vi "Multi-socket save data.vi"(0 "TMN DC\\CAP Data Log File Path":path=path "C:/temp", 1 "SN":T2={"SN_S1"="01", "SN_S2"="02", "SN_S3"="03", "SN_S4"="04", "SN_S5"="05", "SN_S6"="06", "SN_S7"="07", "SN_S8"="08", "SN_S9"="09", "SN_S10"="10", "SN_S11"="11", "SN_S12"="12", "SN_S13"="13", "SN_S14"="14", "SN_S15"="15", "SN_S16"="16"}, 2 "EFUSE":T1={"S1_EFUSE"="0", "S2_EFUSE"="01", "S3_EFUSE"="02", "S4_EFUSE"="04", "S5_EFUSE"="05", "S6_EFUSE"="06", "S7_EFUSE"="07", "S8_EFUSE"="08", "S9_EFUSE"="09", "S10_EFUSE"="10", "S11_EFUSE"="11", "S12_EFUSE"="12", "S13_EFUSE"="13", "S14_EFUSE"="14", "S15_EFUSE"="15", "S16_EFUSE"="16"}, 3 "Lot#":string="WS1033", 4 "Wafer#":string="T4", 5 "File Name":string="Test Data", 7 "error in":errorcluster, 8 "Multi Socket Data Out":string[][](array[string])=[["1", "1", "1", "1", "1", "1", "1", "1", "1", "1", "1", "1", "1", "1", "1", "1", "1", "1", "1", "1", "1", "1", "1", "1", "1", "1", "1", "1", "1", "1", "1", "1", "1", "1", "1", "1", "1", "1", "1", "1", "1", "1", "1", "1", "1", "1", "1", "1", "1", "1", "1", "1", "1", "1", "1", "1", "1", "1", "1", "1", "1", "1", "1", "1", "1", "1", "1", "1", "1", "1", "1", "1", "1", "1", "1", "1", "1", "1", "1", "1", "1", "1", "1"], ["2", "2", "2", "2", "2", "2", "2", "2", "2", "2", "2", "2", "2", "2", "2", "2", "2", "2", "2", "2", "2", "2", "2", "2", "2", "2", "2", "2", "2", "2", "2", "2", "2", "2", "2", "2", "2", "2", "2", "2", "2", "2", "2", "2", "2", "2", "2", "2", "2", "2", "2", "2", "2", "2", "2", "2", "2", "2", "2", "2", "2", "2", "2", "2", "2", "2", "2", "2", "2", "2", "2", "2", "2", "2", "2", "2", "2", "2", "2", "2", "2", "2", "2"], ["3", "3", "3", "3", "3", "3", "3", "3", "3", "3", "3", "3", "3", "3", "3", "3", "3", "3", "3", "3", "3", "3", "3", "3", "3", "3", "3", "3", "3", "3", "3", "3", "3", "3", "3", "3", "3", "3", "3", "3", "3", "3", "3", "3", "3", "3", "3", "3", "3", "3", "3", "3", "3", "3", "3", "3", "3", "3", "3", "3", "3", "3", "3", "3", "3", "3", "3", "3", "3", "3", "3", "3", "3", "3", "3", "3", "3", "3", "3", "3", "3", "3", "3"], ["4", "4", "4", "4", "4", "4", "4", "4", "4", "4", "4", "4", "4", "4", "4", "4", "4", "4", "4", "4", "4", "4", "4", "4", "4", "4", "4", "4", "4", "4", "4", "4", "4", "4", "4", "4", "4", "4", "4", "4", "4", "4", "4", "4", "4", "4", "4", "4", "4", "4", "4", "4", "4", "4", "4", "4", "4", "4", "4", "4", "4", "4", "4", "4", "4", "4", "4", "4", "4", "4", "4", "4", "4", "4", "4", "4", "4", "4", "4", "4", "4", "4", "4"], ["5", "5", "5", "5", "5", "5", "5", "5", "5", "5", "5", "5", "5", "5", "5", "5", "5", "5", "5", "5", "5", "5", "5", "5", "5", "5", "5", "5", "5", "5", "5", "5", "5", "5", "5", "5", "5", "5", "5", "5", "5", "5", "5", "5", "5", "5", "5", "5", "5", "5", "5", "5", "5", "5", "5", "5", "5", "5", "5", "5", "5", "5", "5", "5", "5", "5", "5", "5", "5", "5", "5", "5", "5", "5", "5", "5", "5", "5", "5", "5", "5", "5", "5"], ["6", "6", "6", "6", "6", "6", "6", "6", "6", "6", "6", "6", "6", "6", "6", "6", "6", "6", "6", "6", "6", "6", "6", "6", "6", "6", "6", "6", "6", "6", "6", "6", "6", "6", "6", "6", "6", "6", "6", "6", "6", "6", "6", "6", "6", "6", "6", "6", "6", "6", "6", "6", "6", "6", "6", "6", "6", "6", "6", "6", "6", "6", "6", "6", "6", "6", "6", "6", "6", "6", "6", "6", "6", "6", "6", "6", "6", "6", "6", "6", "6", "6", "6"], ["7", "7", "7", "7", "7", "7", "7", "7", "7", "7", "7", "7", "7", "7", "7", "7", "7", "7", "7", "7", "7", "7", "7", "7", "7", "7", "7", "7", "7", "7", "7", "7", "7", "7", "7", "7", "7", "7", "7", "7", "7", "7", "7", "7", "7", "7", "7", "7", "7", "7", "7", "7", "7", "7", "7", "7", "7", "7", "7", "7", "7", "7", "7", "7", "7", "7", "7", "7", "7", "7", "7", "7", "7", "7", "7", "7", "7", "7", "7", "7", "7", "7", "7"], ["8", "8", "8", "8", "8", "8", "8", "8", "8", "8", "8", "8", "8", "8", "8", "8", "8", "8", "8", "8", "8", "8", "8", "8", "8", "8", "8", "8", "8", "8", "8", "8", "8", "8", "8", "8", "8", "8", "8", "8", "8", "8", "8", "8", "8", "8", "8", "8", "8", "8", "8", "8", "8", "8", "8", "8", "8", "8", "8", "8", "8", "8", "8", "8", "8", "8", "8", "8", "8", "8", "8", "8", "8", "8", "8", "8", "8", "8", "8", "8", "8", "8", "8"], ["9", "9", "9", "9", "9", "9", "9", "9", "9", "9", "9", "9", "9", "9", "9", "9", "9", "9", "9", "9", "9", "9", "9", "9", "9", "9", "9", "9", "9", "9", "9", "9", "9", "9", "9", "9", "9", "9", "9", "9", "9", "9", "9", "9", "9", "9", "9", "9", "9", "9", "9", "9", "9", "9", "9", "9", "9", "9", "9", "9", "9", "9", "9", "9", "9", "9", "9", "9", "9", "9", "9", "9", "9", "9", "9", "9", "9", "9", "9", "9", "9", "9", "9"], ["10", "10", "10", "10", "10", "10", "10", "10", "10", "10", "10", "10", "10", "10", "10", "10", "10", "10", "10", "10", "10", "10", "10", "10", "10", "10", "10", "10", "10", "10", "10", "10", "10", "10", "10", "10", "10", "10", "10", "10", "10", "10", "10", "10", "10", "10", "10", "10", "10", "10", "10", "10", "10", "10", "10", "10", "10", "10", "10", "10", "10", "10", "10", "10", "10", "10", "10", "10", "10", "10", "10", "10", "10", "10", "10", "10", "10", "10", "10", "10", "10", "10", "10"], ["11", "11", "11", "11", "11", "11", "11", "11", "11", "11", "11", "11", "11", "11", "11", "11", "11", "11", "11", "11", "11", "11", "11", "11", "11", "11", "11", "11", "11", "11", "11", "11", "11", "11", "11", "11", "11", "11", "11", "11", "11", "11", "11", "11", "11", "11", "11", "11", "11", "11", "11", "11", "11", "11", "11", "11", "11", "11", "11", "11", "11", "11", "11", "11", "11", "11", "11", "11", "11", "11", "11", "11", "11", "11", "11", "11", "11", "11", "11", "11", "11", "11", "11"], ["12", "12", "12", "12", "12", "12", "12", "12", "12", "12", "12", "12", "12", "12", "12", "12", "12", "12", "12", "12", "12", "12", "12", "12", "12", "12", "12", "12", "12", "12", "12", "12", "12", "12", "12", "12", "12", "12", "12", "12", "12", "12", "12", "12", "12", "12", "12", "12", "12", "12", "12", "12", "12", "12", "12", "12", "12", "12", "12", "12", "12", "12", "12", "12", "12", "12", "12", "12", "12", "12", "12", "12", "12", "12", "12", "12", "12", "12", "12", "12", "12", "12", "12"], ["13", "13", "13", "13", "13", "13", "13", "13", "13", "13", "13", "13", "13", "13", "13", "13", "13", "13", "13", "13", "13", "13", "13", "13", "13", "13", "13", "13", "13", "13", "13", "13", "13", "13", "13", "13", "13", "13", "13", "13", "13", "13", "13", "13", "13", "13", "13", "13", "13", "13", "13", "13", "13", "13", "13", "13", "13", "13", "13", "13", "13", "13", "13", "13", "13", "13", "13", "13", "13", "13", "13", "13", "13", "13", "13", "13", "13", "13", "13", "13", "13", "13", "13"], ["14", "14", "14", "14", "14", "14", "14", "14", "14", "14", "14", "14", "14", "14", "14", "14", "14", "14", "14", "14", "14", "14", "14", "14", "14", "14", "14", "14", "14", "14", "14", "14", "14", "14", "14", "14", "14", "14", "14", "14", "14", "14", "14", "14", "14", "14", "14", "14", "14", "14", "14", "14", "14", "14", "14", "14", "14", "14", "14", "14", "14", "14", "14", "14", "14", "14", "14", "14", "14", "14", "14", "14", "14", "14", "14", "14", "14", "14", "14", "14", "14", "14", "14"], ["15", "15", "15", "15", "15", "15", "15", "15", "15", "15", "15", "15", "15", "15", "15", "15", "15", "15", "15", "15", "15", "15", "15", "15", "15", "15", "15", "15", "15", "15", "15", "15", "15", "15", "15", "15", "15", "15", "15", "15", "15", "15", "15", "15", "15", "15", "15", "15", "15", "15", "15", "15", "15", "15", "15", "15", "15", "15", "15", "15", "15", "15", "15", "15", "15", "15", "15", "15", "15", "15", "15", "15", "15", "15", "15", "15", "15", "15", "15", "15", "15", "15", "15"], ["16", "16", "16", "16", "16", "16", "16", "16", "16", "16", "16", "16", "16", "16", "16", "16", "16", "16", "16", "16", "16", "16", "16", "16", "16", "16", "16", "16", "16", "16", "16", "16", "16", "16", "16", "16", "16", "16", "16", "16", "16", "16", "16", "16", "16", "16", "16", "16", "16", "16", "16", "16", "16", "16", "16", "16", "16", "16", "16", "16", "16", "16", "16", "16", "16", "16", "16", "16", "16", "16", "16", "16", "16", "16", "16", "16", "16", "16", "16", "16", "16", "16", "16"]]) -> (27 "error out":errorcluster)   [LabVIEW 2009]
panel:
  in  "Bin":string="0"
  in  "TP/Comment":cluster{"Test Program":string, "Comment":string}={"Test Program"="Test Data", "Comment"="HD_Cycling"}
  in  "Output":string[][](table)
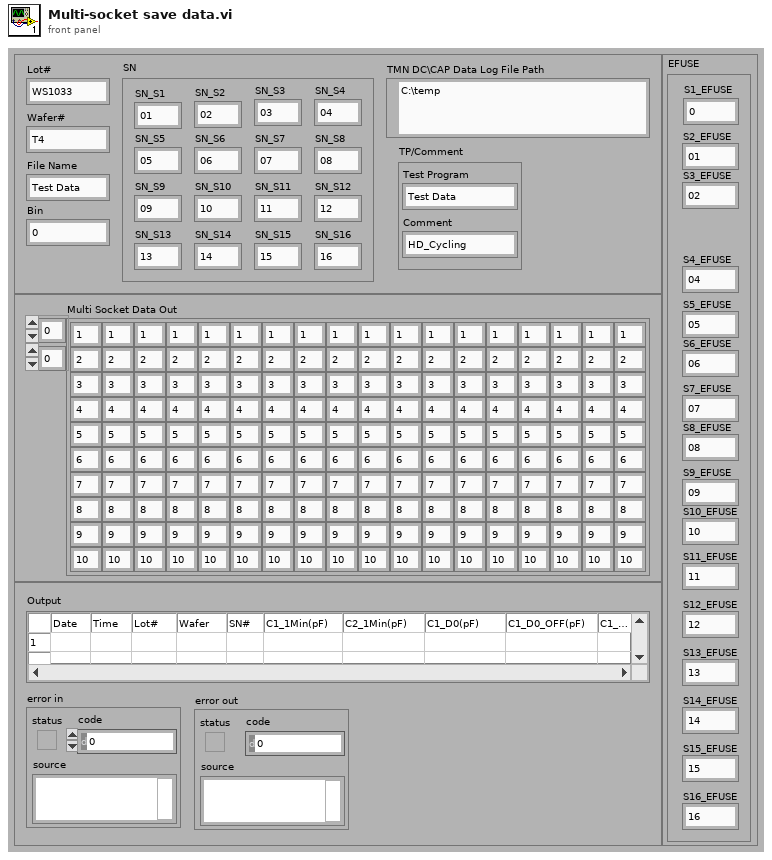
[diagram p1: front panel]
types:
  T1 = cluster{"S1_EFUSE":string, "S2_EFUSE":string, "S3_EFUSE":string, "S4_EFUSE":string, "S5_EFUSE":string, "S6_EFUSE":string, "S7_EFUSE":string, "S8_EFUSE":string, "S9_EFUSE":string, "S10_EFUSE":string, "S11_EFUSE":string, "S12_EFUSE":string, "S13_EFUSE":string, "S14_EFUSE":string, "S15_EFUSE":string, "S16_EFUSE":string}
  T2 = cluster{"SN_S1":string, "SN_S2":string, "SN_S3":string, "SN_S4":string, "SN_S5":string, "SN_S6":string, "SN_S7":string, "SN_S8":string, "SN_S9":string, "SN_S10":string, "SN_S11":string, "SN_S12":string, "SN_S13":string, "SN_S14":string, "SN_S15":string, "SN_S16":string}
  T3 = enum16{"open", "replace", "create", "open or create", "replace or create", "replace or create with confirmation"}
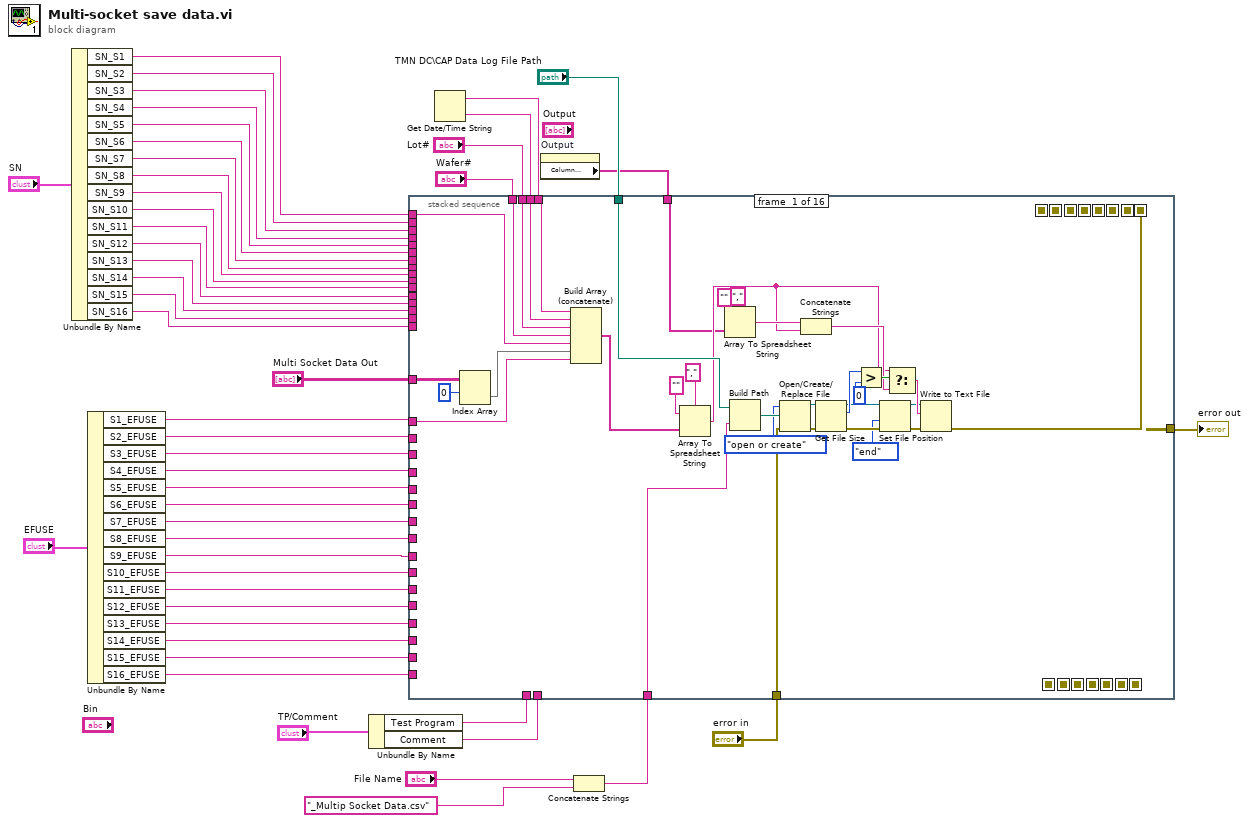
[diagram p0: block diagram]
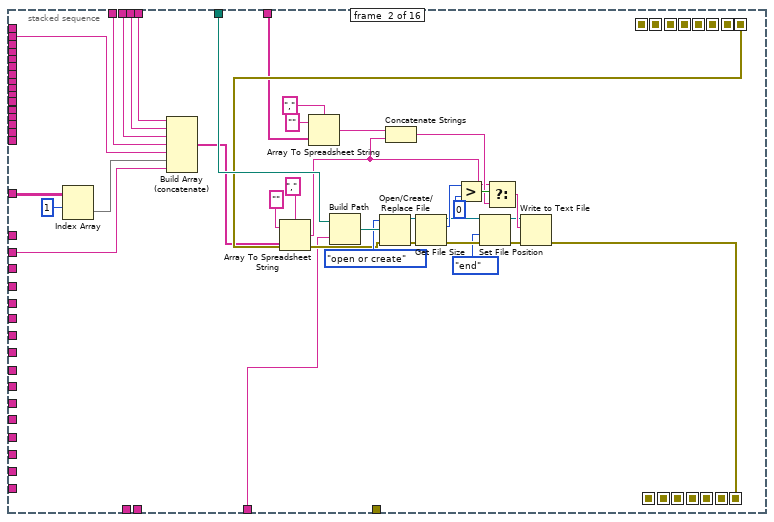
[diagram p2: hidden frame]
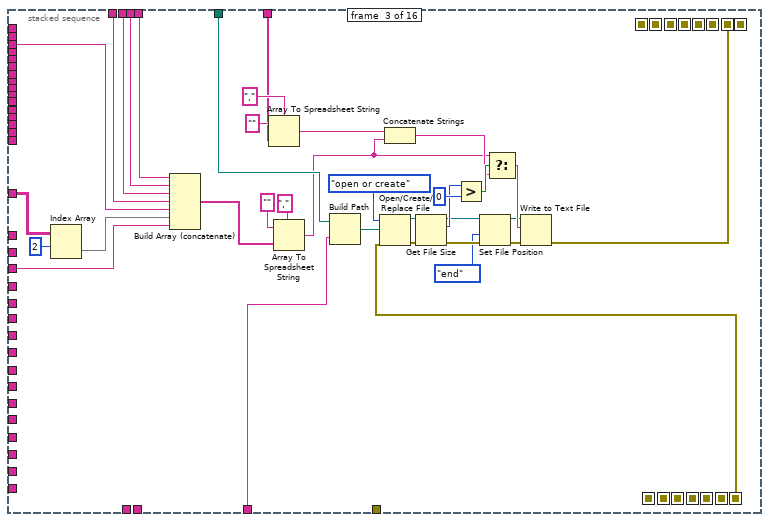
[diagram p3: hidden frame]
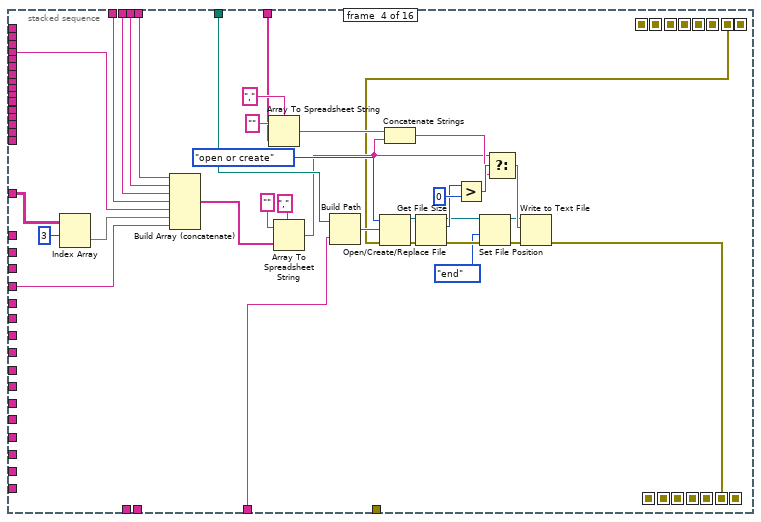
[diagram p4: hidden frame]
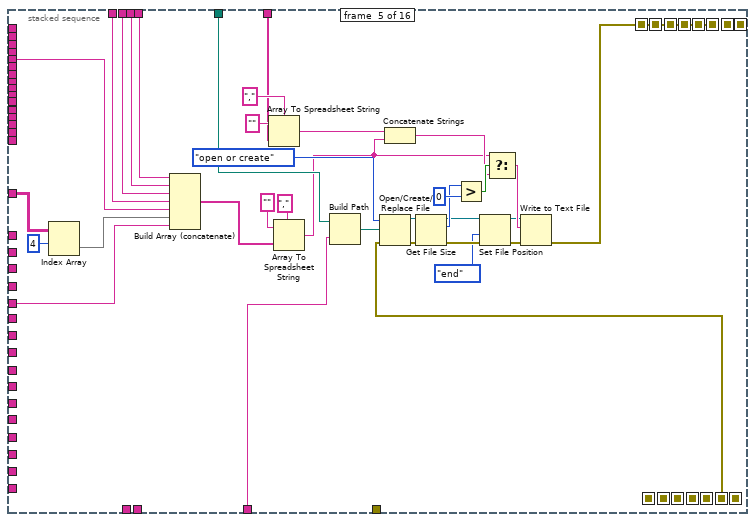
[diagram p5: hidden frame]
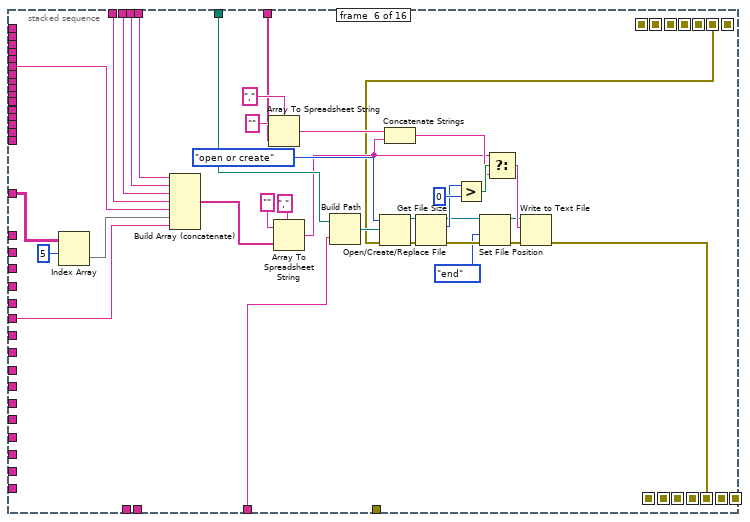
[diagram p6: hidden frame]
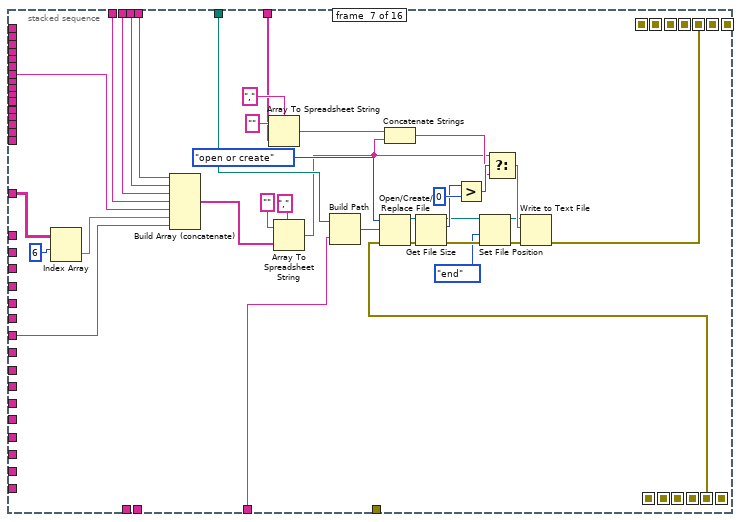
[diagram p7: hidden frame]
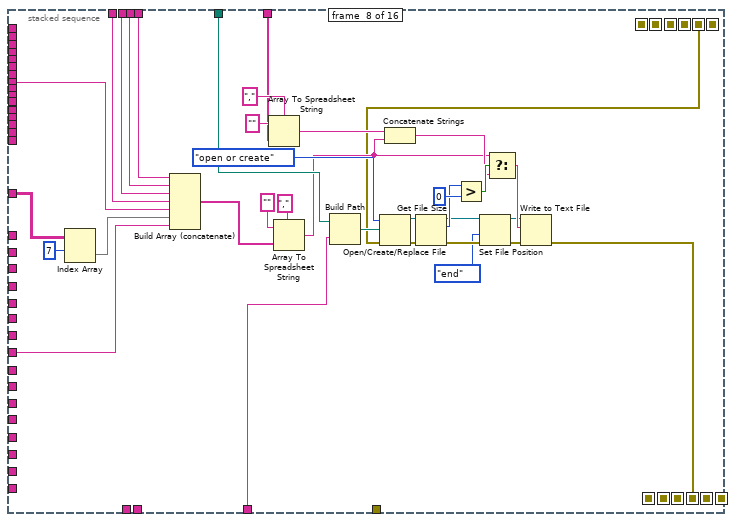
[diagram p8: hidden frame]
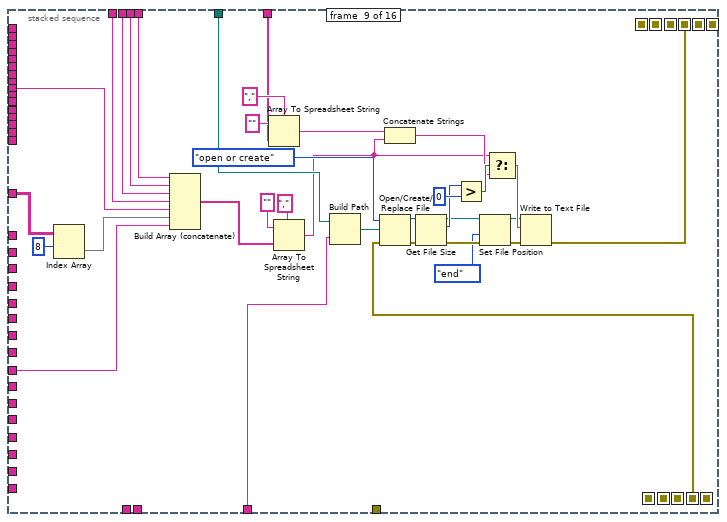
[diagram p9: hidden frame]
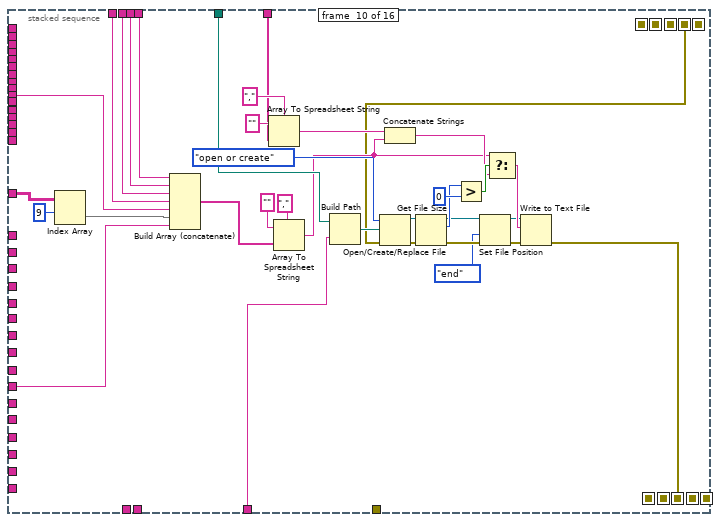
[diagram p10: hidden frame]
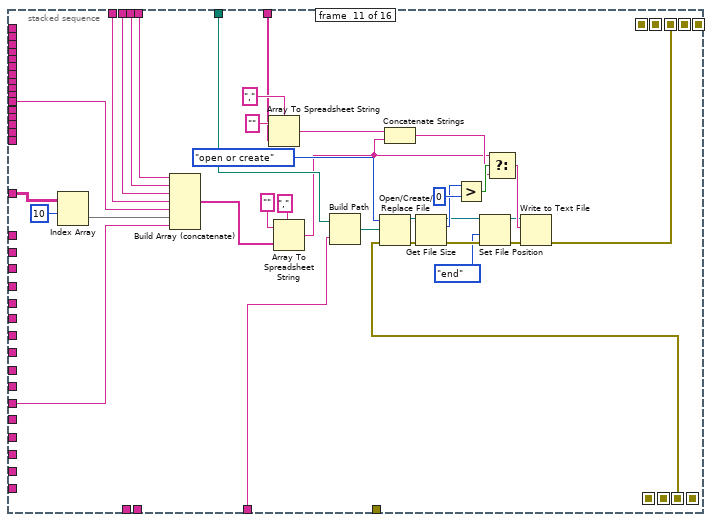
[diagram p11: hidden frame]
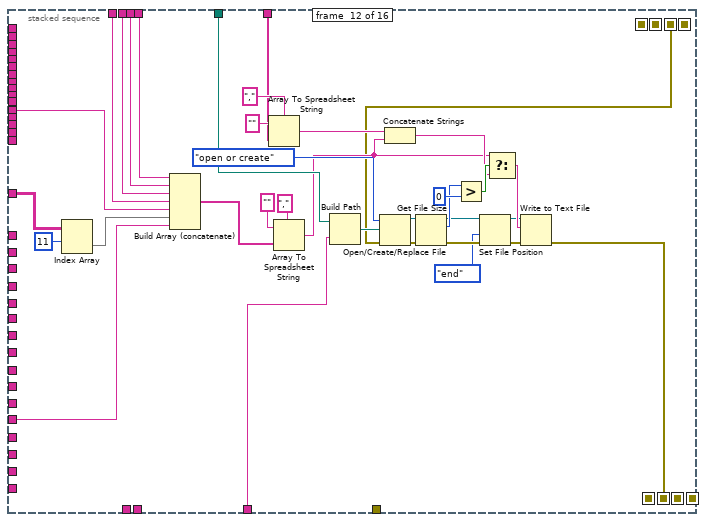
[diagram p12: hidden frame]
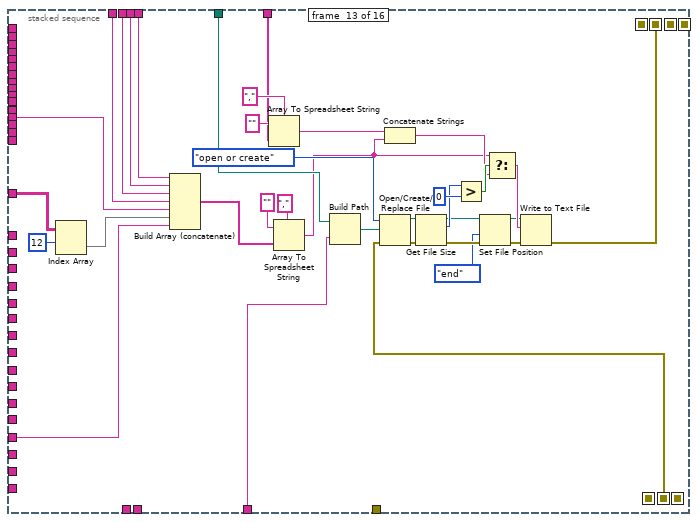
[diagram p13: hidden frame]
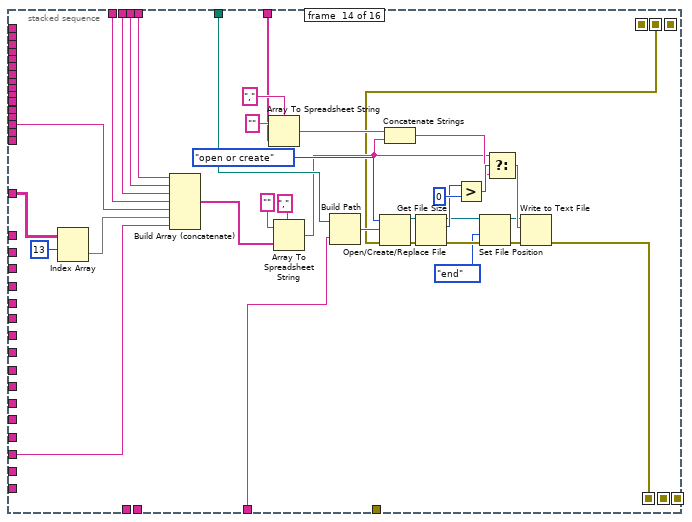
[diagram p14: hidden frame]
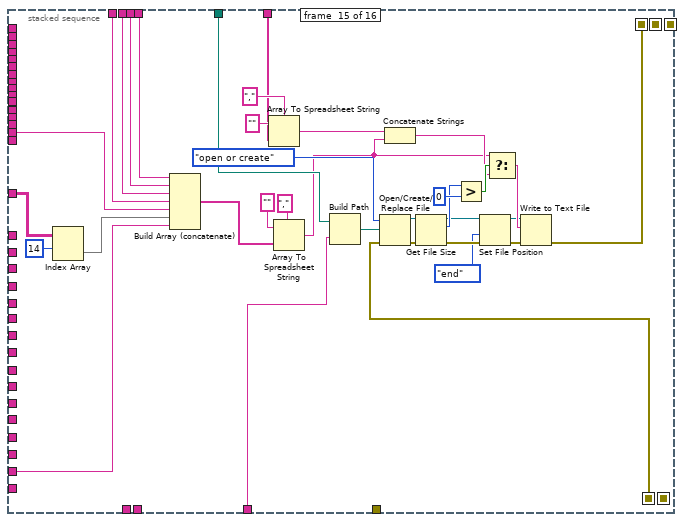
[diagram p15: hidden frame]
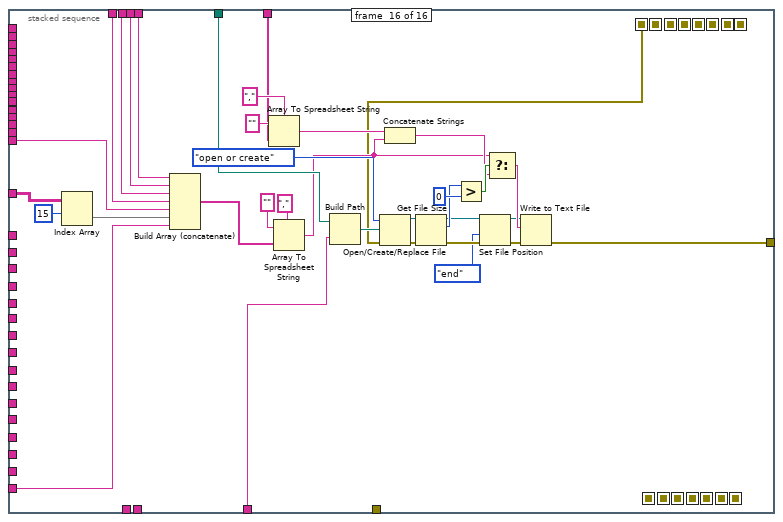
[diagram p16: hidden frame]
diagram:
  n1 = Unbundle By Name("SN") -> ("SN_S1"=w40:string, "SN_S2"=w39:string, "SN_S3"=w38:string, "SN_S4"=w34:string, "SN_S5"=w33:string, "SN_S6"=w32:string, "SN_S7"=w31:string, "SN_S8"=w30:string, "SN_S9"=w29:string, "SN_S10"=w28:string, "SN_S11"=w27:string, "SN_S12"=w26:string, "SN_S13"=w25:string, "SN_S14"=w24:string, "SN_S15"=w23:string, "SN_S16"=w22:string)
  n2 = Unbundle By Name("EFUSE") -> ("S1_EFUSE"=w19:string, "S2_EFUSE"=w18:string, "S3_EFUSE"=w17:string, "S4_EFUSE"=w16:string, "S5_EFUSE"=w15:string, "S6_EFUSE"=w14:string, "S7_EFUSE"=w13:string, "S8_EFUSE"=w12:string, "S9_EFUSE"=w11:string, "S10_EFUSE"=w10:string, "S11_EFUSE"=w9:string, "S12_EFUSE"=w8:string, "S13_EFUSE"=w7:string, "S14_EFUSE"=w6:string, "S15_EFUSE"=w5:string, "S16_EFUSE"=w4:string)
  n3 = Unbundle By Name("TP/Comment") -> ("Test Program"=w36:string, "Comment"=w35:string)
  n4 = Get Date/Time String() -> (date string=w46:string, time string=w45:string)  [unwired: 3 in]
  n5 = property on="Output" class="Tbl (strict)"() -> ("Column Headers[]"=w47:string[])  [unwired: 2 in, 2 out]
  n6 = Concatenate Strings("File Name", "_Multip Socket Data.csv" ("string")) -> (w1:string)
  n7 = stacked-sequence {
    seq-local: [w62 _ _ _ _ _ _ _ _ _ _ _ _ _ _ _] -> [_ w98 _ _ _ _ _ _ _ _ _ _ _ _ _ _]
    seq-local: [_ w97 _ _ _ _ _ _ _ _ _ _ _ _ _ _] -> [_ _ w133 _ _ _ _ _ _ _ _ _ _ _ _ _]
    seq-local: [_ _ w126 _ _ _ _ _ _ _ _ _ _ _ _ _] -> [_ _ _ w162 _ _ _ _ _ _ _ _ _ _ _ _]
    seq-local: [_ _ _ w161 _ _ _ _ _ _ _ _ _ _ _ _] -> [_ _ _ _ w197 _ _ _ _ _ _ _ _ _ _ _]
    seq-local: [_ _ _ _ w196 _ _ _ _ _ _ _ _ _ _ _] -> [_ _ _ _ _ w232 _ _ _ _ _ _ _ _ _ _]
    seq-local: [_ _ _ _ _ w231 _ _ _ _ _ _ _ _ _ _] -> [_ _ _ _ _ _ w267 _ _ _ _ _ _ _ _ _]
    seq-local: [_ _ _ _ _ _ w266 _ _ _ _ _ _ _ _ _] -> [_ _ _ _ _ _ _ w302 _ _ _ _ _ _ _ _]
    seq-local: [_ _ _ _ _ _ _ w301 _ _ _ _ _ _ _ _] -> [_ _ _ _ _ _ _ _ w337 _ _ _ _ _ _ _]
    seq-local: [_ _ _ _ _ _ _ _ w336 _ _ _ _ _ _ _] -> [_ _ _ _ _ _ _ _ _ w372 _ _ _ _ _ _]
    seq-local: [_ _ _ _ _ _ _ _ _ w371 _ _ _ _ _ _] -> [_ _ _ _ _ _ _ _ _ _ w407 _ _ _ _ _]
    seq-local: [_ _ _ _ _ _ _ _ _ _ w406 _ _ _ _ _] -> [_ _ _ _ _ _ _ _ _ _ _ w442 _ _ _ _]
    seq-local: [_ _ _ _ _ _ _ _ _ _ _ w441 _ _ _ _] -> [_ _ _ _ _ _ _ _ _ _ _ _ w477 _ _ _]
    seq-local: [_ _ _ _ _ _ _ _ _ _ _ _ w476 _ _ _] -> [_ _ _ _ _ _ _ _ _ _ _ _ _ w512 _ _]
    seq-local: [_ _ _ _ _ _ _ _ _ _ _ _ _ w511 _ _] -> [_ _ _ _ _ _ _ _ _ _ _ _ _ _ w547 _]
    seq-local: [_ _ _ _ _ _ _ _ _ _ _ _ _ _ w546 _] -> [_ _ _ _ _ _ _ _ _ _ _ _ _ _ _ w582]
    tunnel: "TMN DC\\CAP Data Log File Path" -> [w65 w100 w135 w170 w205 w240 w275 w310 w345 w380 w415 w450 w485 w520 w555 w590]
    tunnel: "error in" -> [w63 _ _ _ _ _ _ _ _ _ _ _ _ _ _ _]
    tunnel: [_ _ _ _ _ _ _ _ _ _ _ _ _ _ _ w581] -> w48
    tunnel: w47 -> [w61 w96 w132 w168 w203 w238 w273 w308 w343 w378 w413 w448 w483 w518 w553 w588]
    tunnel: w46 -> [w59 w95 w130 w166 w201 w236 w271 w306 w341 w376 w411 w446 w481 w516 w551 w586]
    tunnel: w45 -> [w58 w91 w129 w165 w200 w235 w270 w305 w340 w375 w410 w445 w480 w515 w550 w585]
    tunnel: "Lot#" -> [w57 w93 w128 w164 w199 w234 w269 w304 w339 w374 w409 w444 w479 w514 w549 w584]
    tunnel: "Wafer#" -> [w56 w92 w127 w163 w198 w233 w268 w303 w338 w373 w408 w443 w478 w513 w548 w583]
    tunnel: w40 -> [w55 _ _ _ _ _ _ _ _ _ _ _ _ _ _ _]
    tunnel: w39 -> [_ w90 _ _ _ _ _ _ _ _ _ _ _ _ _ _]
    tunnel: w38 -> [_ _ w125 _ _ _ _ _ _ _ _ _ _ _ _ _]
    tunnel: w36 -> [_ _ _ _ _ _ _ _ _ _ _ _ _ _ _ _]
    tunnel: w35 -> [_ _ _ _ _ _ _ _ _ _ _ _ _ _ _ _]
    tunnel: w34 -> [_ _ _ w160 _ _ _ _ _ _ _ _ _ _ _ _]
    tunnel: w33 -> [_ _ _ _ w195 _ _ _ _ _ _ _ _ _ _ _]
    tunnel: w32 -> [_ _ _ _ _ w230 _ _ _ _ _ _ _ _ _ _]
    tunnel: w31 -> [_ _ _ _ _ _ w265 _ _ _ _ _ _ _ _ _]
    tunnel: w30 -> [_ _ _ _ _ _ _ w300 _ _ _ _ _ _ _ _]
    tunnel: w29 -> [_ _ _ _ _ _ _ _ w335 _ _ _ _ _ _ _]
    tunnel: w28 -> [_ _ _ _ _ _ _ _ _ w370 _ _ _ _ _ _]
    tunnel: w27 -> [_ _ _ _ _ _ _ _ _ _ w405 _ _ _ _ _]
    tunnel: w26 -> [_ _ _ _ _ _ _ _ _ _ _ w440 _ _ _ _]
    tunnel: w25 -> [_ _ _ _ _ _ _ _ _ _ _ _ w475 _ _ _]
    tunnel: w24 -> [_ _ _ _ _ _ _ _ _ _ _ _ _ w510 _ _]
    tunnel: w23 -> [_ _ _ _ _ _ _ _ _ _ _ _ _ _ w545 _]
    tunnel: w22 -> [_ _ _ _ _ _ _ _ _ _ _ _ _ _ _ w580]
    tunnel: "Multi Socket Data Out" -> [w53 w89 w124 w158 w192 w229 w263 w298 w333 w368 w403 w438 w473 w507 w543 w578]
    tunnel: w19 -> [w51 _ _ _ _ _ _ _ _ _ _ _ _ _ _ _]
    tunnel: w18 -> [_ w86 _ _ _ _ _ _ _ _ _ _ _ _ _ _]
    tunnel: w17 -> [_ _ w121 _ _ _ _ _ _ _ _ _ _ _ _ _]
    tunnel: w16 -> [_ _ _ w156 _ _ _ _ _ _ _ _ _ _ _ _]
    tunnel: w15 -> [_ _ _ _ w191 _ _ _ _ _ _ _ _ _ _ _]
    tunnel: w14 -> [_ _ _ _ _ w226 _ _ _ _ _ _ _ _ _ _]
    tunnel: w13 -> [_ _ _ _ _ _ w261 _ _ _ _ _ _ _ _ _]
    tunnel: w12 -> [_ _ _ _ _ _ _ w296 _ _ _ _ _ _ _ _]
    tunnel: w11 -> [_ _ _ _ _ _ _ _ w331 _ _ _ _ _ _ _]
    tunnel: w10 -> [_ _ _ _ _ _ _ _ _ w366 _ _ _ _ _ _]
    tunnel: w9 -> [_ _ _ _ _ _ _ _ _ _ w401 _ _ _ _ _]
    tunnel: w8 -> [_ _ _ _ _ _ _ _ _ _ _ w436 _ _ _ _]
    tunnel: w7 -> [_ _ _ _ _ _ _ _ _ _ _ _ w471 _ _ _]
    tunnel: w6 -> [_ _ _ _ _ _ _ _ _ _ _ _ _ w506 _ _]
    tunnel: w5 -> [_ _ _ _ _ _ _ _ _ _ _ _ _ _ w541 _]
    tunnel: w4 -> [_ _ _ _ _ _ _ _ _ _ _ _ _ _ _ w576]
    tunnel: w1 -> [w50 w85 w120 w155 w190 w225 w260 w295 w330 w365 w400 w435 w470 w505 w540 w575]
    frame #0 {
      n8 = Index Array(array=w53, index (row)=0) -> (element=w52:string[])  [unwired: 1 in]
      n9 = Build Array (concatenate)(w59, w58, w57, w56, w55, w52, w51) -> (w60:string[])
      n10 = Array To Spreadsheet String(delimiter (Tab)=",", array=w60, 3:"" ("format string")) -> (spreadsheet string=w64:string)
      n11 = Array To Spreadsheet String(delimiter (Tab)=",", array=w61, 3:"" ("format string")) -> (spreadsheet string=w67:string)
      n12 = Build Path(base path=w65, name or relative path=w50) -> (appended path=w79:path)
      n13 = Open/Create/Replace File(file path (use dialog)=w79, error in=w63, operation (0:open)=T3."open or create") -> (refnum out=w77:refnum<file>, error out=w80:errorcluster)  [unwired: 4 out]
      n14 = Concatenate Strings(w67, w64) -> (w66:string)
      n15 = Get File Size(file=w77, error in=w80) -> (refnum out=w72:refnum<file>, size (in bytes)=w76:i64, 0:w74:errorcluster)
      n16 = Greater?(x=w76, y=i64 0) -> (0:w81:bool)
      n17 = Set File Position(refnum=w72, from (0:start)=enum16{"start", "end", "current"}."end", error in=w74) -> (refnum out=w71:refnum<file>, error out=w73:errorcluster)  [unwired: 1 out]
      n18 = Select(t=w64, s=w81, f=w66) -> (s? t:f=w78:string)
      n19 = Write to Text File(file (use dialog)=w71, text=w78, error in=w73) -> (error out=w62:errorcluster)  [unwired: 3 out]
    }
    frame #1 {
      n20 = Index Array(array=w89, index (row)=1) -> (element=w87:string[])  [unwired: 1 in]
      n21 = Build Array (concatenate)(w95, w91, w93, w92, w90, w87, w86) -> (w94:string[])
      n22 = Array To Spreadsheet String(delimiter (Tab)=",", array=w94, 3:"" ("format string")) -> (spreadsheet string=w99:string)
      n23 = Array To Spreadsheet String(delimiter (Tab)=",", array=w96, 3:"" ("format string")) -> (spreadsheet string=w102:string)
      n24 = Build Path(base path=w100, name or relative path=w85) -> (appended path=w114:path)
      n25 = Open/Create/Replace File(file path (use dialog)=w114, error in=w98, operation (0:open)=T3."open or create") -> (refnum out=w112:refnum<file>, error out=w115:errorcluster)  [unwired: 4 out]
      n26 = Concatenate Strings(w102, w99) -> (w101:string)
      n27 = Get File Size(file=w112, error in=w115) -> (refnum out=w107:refnum<file>, size (in bytes)=w111:i64, 0:w109:errorcluster)
      n28 = Greater?(x=w111, y=i64 0) -> (0:w116:bool)
      n29 = Set File Position(refnum=w107, from (0:start)=enum16{"start", "end", "current"}."end", error in=w109) -> (refnum out=w106:refnum<file>, error out=w108:errorcluster)  [unwired: 1 out]
      n30 = Select(t=w99, s=w116, f=w101) -> (s? t:f=w113:string)
      n31 = Write to Text File(file (use dialog)=w106, text=w113, error in=w108) -> (error out=w97:errorcluster)  [unwired: 3 out]
    }
    frame #2 {
      n32 = Index Array(array=w124, index (row)=2) -> (element=w122:string[])  [unwired: 1 in]
      n33 = Build Array (concatenate)(w130, w129, w128, w127, w125, w122, w121) -> (w131:string[])
      n34 = Array To Spreadsheet String(delimiter (Tab)=",", array=w132, 3:"" ("format string")) -> (spreadsheet string=w137:string)
      n35 = Array To Spreadsheet String(delimiter (Tab)=",", array=w131, 3:"" ("format string")) -> (spreadsheet string=w134:string)
      n36 = Build Path(base path=w135, name or relative path=w120) -> (appended path=w149:path)
      n37 = Open/Create/Replace File(file path (use dialog)=w149, error in=w133, operation (0:open)=T3."open or create") -> (refnum out=w147:refnum<file>, error out=w150:errorcluster)  [unwired: 4 out]
      n38 = Concatenate Strings(w137, w134) -> (w136:string)
      n39 = Get File Size(file=w147, error in=w150) -> (refnum out=w142:refnum<file>, size (in bytes)=w146:i64, 0:w144:errorcluster)
      n40 = Greater?(x=w146, y=i64 0) -> (0:w151:bool)
      n41 = Set File Position(refnum=w142, from (0:start)=enum16{"start", "end", "current"}."end", error in=w144) -> (refnum out=w141:refnum<file>, error out=w143:errorcluster)  [unwired: 1 out]
      n42 = Select(t=w134, s=w151, f=w136) -> (s? t:f=w148:string)
      n43 = Write to Text File(file (use dialog)=w141, text=w148, error in=w143) -> (error out=w126:errorcluster)  [unwired: 3 out]
    }
    frame #3 {
      n44 = Index Array(array=w158, index (row)=3) -> (element=w159:string[])  [unwired: 1 in]
      n45 = Build Array (concatenate)(w166, w165, w164, w163, w160, w159, w156) -> (w167:string[])
      n46 = Array To Spreadsheet String(delimiter (Tab)=",", array=w168, 3:"" ("format string")) -> (spreadsheet string=w172:string)
      n47 = Array To Spreadsheet String(delimiter (Tab)=",", array=w167, 3:"" ("format string")) -> (spreadsheet string=w169:string)
      n48 = Build Path(base path=w170, name or relative path=w155) -> (appended path=w184:path)
      n49 = Open/Create/Replace File(file path (use dialog)=w184, error in=w162, operation (0:open)=T3."open or create") -> (refnum out=w182:refnum<file>, error out=w185:errorcluster)  [unwired: 4 out]
      n50 = Concatenate Strings(w172, w169) -> (w171:string)
      n51 = Get File Size(file=w182, error in=w185) -> (refnum out=w177:refnum<file>, size (in bytes)=w181:i64, 0:w179:errorcluster)
      n52 = Greater?(x=w181, y=i64 0) -> (0:w186:bool)
      n53 = Set File Position(refnum=w177, from (0:start)=enum16{"start", "end", "current"}."end", error in=w179) -> (refnum out=w176:refnum<file>, error out=w178:errorcluster)  [unwired: 1 out]
      n54 = Select(t=w169, s=w186, f=w171) -> (s? t:f=w183:string)
      n55 = Write to Text File(file (use dialog)=w176, text=w183, error in=w178) -> (error out=w161:errorcluster)  [unwired: 3 out]
    }
    frame #4 {
      n56 = Index Array(array=w192, index (row)=4) -> (element=w193:string[])  [unwired: 1 in]
      n57 = Build Array (concatenate)(w201, w200, w199, w198, w195, w193, w191) -> (w202:string[])
      n58 = Array To Spreadsheet String(delimiter (Tab)=",", array=w203, 3:"" ("format string")) -> (spreadsheet string=w207:string)
      n59 = Array To Spreadsheet String(delimiter (Tab)=",", array=w202, 3:"" ("format string")) -> (spreadsheet string=w204:string)
      n60 = Build Path(base path=w205, name or relative path=w190) -> (appended path=w219:path)
      n61 = Open/Create/Replace File(file path (use dialog)=w219, error in=w197, operation (0:open)=T3."open or create") -> (refnum out=w217:refnum<file>, error out=w220:errorcluster)  [unwired: 4 out]
      n62 = Concatenate Strings(w207, w204) -> (w206:string)
      n63 = Get File Size(file=w217, error in=w220) -> (refnum out=w212:refnum<file>, size (in bytes)=w216:i64, 0:w214:errorcluster)
      n64 = Greater?(x=w216, y=i64 0) -> (0:w221:bool)
      n65 = Set File Position(refnum=w212, from (0:start)=enum16{"start", "end", "current"}."end", error in=w214) -> (refnum out=w211:refnum<file>, error out=w213:errorcluster)  [unwired: 1 out]
      n66 = Select(t=w204, s=w221, f=w206) -> (s? t:f=w218:string)
      n67 = Write to Text File(file (use dialog)=w211, text=w218, error in=w213) -> (error out=w196:errorcluster)  [unwired: 3 out]
    }
    frame #5 {
      n68 = Index Array(array=w229, index (row)=5) -> (element=w228:string[])  [unwired: 1 in]
      n69 = Build Array (concatenate)(w236, w235, w234, w233, w230, w228, w226) -> (w237:string[])
      n70 = Array To Spreadsheet String(delimiter (Tab)=",", array=w238, 3:"" ("format string")) -> (spreadsheet string=w242:string)
      n71 = Array To Spreadsheet String(delimiter (Tab)=",", array=w237, 3:"" ("format string")) -> (spreadsheet string=w239:string)
      n72 = Build Path(base path=w240, name or relative path=w225) -> (appended path=w254:path)
      n73 = Open/Create/Replace File(file path (use dialog)=w254, error in=w232, operation (0:open)=T3."open or create") -> (refnum out=w252:refnum<file>, error out=w255:errorcluster)  [unwired: 4 out]
      n74 = Concatenate Strings(w242, w239) -> (w241:string)
      n75 = Get File Size(file=w252, error in=w255) -> (refnum out=w247:refnum<file>, size (in bytes)=w251:i64, 0:w249:errorcluster)
      n76 = Greater?(x=w251, y=i64 0) -> (0:w256:bool)
      n77 = Set File Position(refnum=w247, from (0:start)=enum16{"start", "end", "current"}."end", error in=w249) -> (refnum out=w246:refnum<file>, error out=w248:errorcluster)  [unwired: 1 out]
      n78 = Select(t=w239, s=w256, f=w241) -> (s? t:f=w253:string)
      n79 = Write to Text File(file (use dialog)=w246, text=w253, error in=w248) -> (error out=w231:errorcluster)  [unwired: 3 out]
    }
    frame #6 {
      n80 = Index Array(array=w263, index (row)=6) -> (element=w262:string[])  [unwired: 1 in]
      n81 = Build Array (concatenate)(w271, w270, w269, w268, w265, w262, w261) -> (w272:string[])
      n82 = Array To Spreadsheet String(delimiter (Tab)=",", array=w273, 3:"" ("format string")) -> (spreadsheet string=w277:string)
      n83 = Array To Spreadsheet String(delimiter (Tab)=",", array=w272, 3:"" ("format string")) -> (spreadsheet string=w274:string)
      n84 = Build Path(base path=w275, name or relative path=w260) -> (appended path=w289:path)
      n85 = Open/Create/Replace File(file path (use dialog)=w289, error in=w267, operation (0:open)=T3."open or create") -> (refnum out=w287:refnum<file>, error out=w290:errorcluster)  [unwired: 4 out]
      n86 = Concatenate Strings(w277, w274) -> (w276:string)
      n87 = Get File Size(file=w287, error in=w290) -> (refnum out=w282:refnum<file>, size (in bytes)=w286:i64, 0:w284:errorcluster)
      n88 = Greater?(x=w286, y=i64 0) -> (0:w291:bool)
      n89 = Set File Position(refnum=w282, from (0:start)=enum16{"start", "end", "current"}."end", error in=w284) -> (refnum out=w281:refnum<file>, error out=w283:errorcluster)  [unwired: 1 out]
      n90 = Select(t=w274, s=w291, f=w276) -> (s? t:f=w288:string)
      n91 = Write to Text File(file (use dialog)=w281, text=w288, error in=w283) -> (error out=w266:errorcluster)  [unwired: 3 out]
    }
    frame #7 {
      n92 = Index Array(array=w298, index (row)=7) -> (element=w297:string[])  [unwired: 1 in]
      n93 = Build Array (concatenate)(w306, w305, w304, w303, w300, w297, w296) -> (w307:string[])
      n94 = Array To Spreadsheet String(delimiter (Tab)=",", array=w308, 3:"" ("format string")) -> (spreadsheet string=w312:string)
      n95 = Array To Spreadsheet String(delimiter (Tab)=",", array=w307, 3:"" ("format string")) -> (spreadsheet string=w309:string)
      n96 = Build Path(base path=w310, name or relative path=w295) -> (appended path=w324:path)
      n97 = Open/Create/Replace File(file path (use dialog)=w324, error in=w302, operation (0:open)=T3."open or create") -> (refnum out=w322:refnum<file>, error out=w325:errorcluster)  [unwired: 4 out]
      n98 = Concatenate Strings(w312, w309) -> (w311:string)
      n99 = Get File Size(file=w322, error in=w325) -> (refnum out=w317:refnum<file>, size (in bytes)=w321:i64, 0:w319:errorcluster)
      n100 = Greater?(x=w321, y=i64 0) -> (0:w326:bool)
      n101 = Set File Position(refnum=w317, from (0:start)=enum16{"start", "end", "current"}."end", error in=w319) -> (refnum out=w316:refnum<file>, error out=w318:errorcluster)  [unwired: 1 out]
      n102 = Select(t=w309, s=w326, f=w311) -> (s? t:f=w323:string)
      n103 = Write to Text File(file (use dialog)=w316, text=w323, error in=w318) -> (error out=w301:errorcluster)  [unwired: 3 out]
    }
    frame #8 {
      n104 = Index Array(array=w333, index (row)=8) -> (element=w332:string[])  [unwired: 1 in]
      n105 = Build Array (concatenate)(w341, w340, w339, w338, w335, w332, w331) -> (w342:string[])
      n106 = Array To Spreadsheet String(delimiter (Tab)=",", array=w343, 3:"" ("format string")) -> (spreadsheet string=w347:string)
      n107 = Array To Spreadsheet String(delimiter (Tab)=",", array=w342, 3:"" ("format string")) -> (spreadsheet string=w344:string)
      n108 = Build Path(base path=w345, name or relative path=w330) -> (appended path=w359:path)
      n109 = Open/Create/Replace File(file path (use dialog)=w359, error in=w337, operation (0:open)=T3."open or create") -> (refnum out=w357:refnum<file>, error out=w360:errorcluster)  [unwired: 4 out]
      n110 = Concatenate Strings(w347, w344) -> (w346:string)
      n111 = Get File Size(file=w357, error in=w360) -> (refnum out=w352:refnum<file>, size (in bytes)=w356:i64, 0:w354:errorcluster)
      n112 = Greater?(x=w356, y=i64 0) -> (0:w361:bool)
      n113 = Set File Position(refnum=w352, from (0:start)=enum16{"start", "end", "current"}."end", error in=w354) -> (refnum out=w351:refnum<file>, error out=w353:errorcluster)  [unwired: 1 out]
      n114 = Select(t=w344, s=w361, f=w346) -> (s? t:f=w358:string)
      n115 = Write to Text File(file (use dialog)=w351, text=w358, error in=w353) -> (error out=w336:errorcluster)  [unwired: 3 out]
    }
    frame #9 {
      n116 = Index Array(array=w368, index (row)=9) -> (element=w367:string[])  [unwired: 1 in]
      n117 = Build Array (concatenate)(w376, w375, w374, w373, w370, w367, w366) -> (w377:string[])
      n118 = Array To Spreadsheet String(delimiter (Tab)=",", array=w378, 3:"" ("format string")) -> (spreadsheet string=w382:string)
      n119 = Array To Spreadsheet String(delimiter (Tab)=",", array=w377, 3:"" ("format string")) -> (spreadsheet string=w379:string)
      n120 = Build Path(base path=w380, name or relative path=w365) -> (appended path=w394:path)
      n121 = Open/Create/Replace File(file path (use dialog)=w394, error in=w372, operation (0:open)=T3."open or create") -> (refnum out=w392:refnum<file>, error out=w395:errorcluster)  [unwired: 4 out]
      n122 = Concatenate Strings(w382, w379) -> (w381:string)
      n123 = Get File Size(file=w392, error in=w395) -> (refnum out=w387:refnum<file>, size (in bytes)=w391:i64, 0:w389:errorcluster)
      n124 = Greater?(x=w391, y=i64 0) -> (0:w396:bool)
      n125 = Set File Position(refnum=w387, from (0:start)=enum16{"start", "end", "current"}."end", error in=w389) -> (refnum out=w386:refnum<file>, error out=w388:errorcluster)  [unwired: 1 out]
      n126 = Select(t=w379, s=w396, f=w381) -> (s? t:f=w393:string)
      n127 = Write to Text File(file (use dialog)=w386, text=w393, error in=w388) -> (error out=w371:errorcluster)  [unwired: 3 out]
    }
    frame #10 {
      n128 = Index Array(array=w403, index (row)=10) -> (element=w402:string[])  [unwired: 1 in]
      n129 = Build Array (concatenate)(w411, w410, w409, w408, w405, w402, w401) -> (w412:string[])
      n130 = Array To Spreadsheet String(delimiter (Tab)=",", array=w413, 3:"" ("format string")) -> (spreadsheet string=w417:string)
      n131 = Array To Spreadsheet String(delimiter (Tab)=",", array=w412, 3:"" ("format string")) -> (spreadsheet string=w414:string)
      n132 = Build Path(base path=w415, name or relative path=w400) -> (appended path=w429:path)
      n133 = Open/Create/Replace File(file path (use dialog)=w429, error in=w407, operation (0:open)=T3."open or create") -> (refnum out=w427:refnum<file>, error out=w430:errorcluster)  [unwired: 4 out]
      n134 = Concatenate Strings(w417, w414) -> (w416:string)
      n135 = Get File Size(file=w427, error in=w430) -> (refnum out=w422:refnum<file>, size (in bytes)=w426:i64, 0:w424:errorcluster)
      n136 = Greater?(x=w426, y=i64 0) -> (0:w431:bool)
      n137 = Set File Position(refnum=w422, from (0:start)=enum16{"start", "end", "current"}."end", error in=w424) -> (refnum out=w421:refnum<file>, error out=w423:errorcluster)  [unwired: 1 out]
      n138 = Select(t=w414, s=w431, f=w416) -> (s? t:f=w428:string)
      n139 = Write to Text File(file (use dialog)=w421, text=w428, error in=w423) -> (error out=w406:errorcluster)  [unwired: 3 out]
    }
    frame #11 {
      n140 = Index Array(array=w438, index (row)=11) -> (element=w437:string[])  [unwired: 1 in]
      n141 = Build Array (concatenate)(w446, w445, w444, w443, w440, w437, w436) -> (w447:string[])
      n142 = Array To Spreadsheet String(delimiter (Tab)=",", array=w448, 3:"" ("format string")) -> (spreadsheet string=w452:string)
      n143 = Array To Spreadsheet String(delimiter (Tab)=",", array=w447, 3:"" ("format string")) -> (spreadsheet string=w449:string)
      n144 = Build Path(base path=w450, name or relative path=w435) -> (appended path=w464:path)
      n145 = Open/Create/Replace File(file path (use dialog)=w464, error in=w442, operation (0:open)=T3."open or create") -> (refnum out=w462:refnum<file>, error out=w465:errorcluster)  [unwired: 4 out]
      n146 = Concatenate Strings(w452, w449) -> (w451:string)
      n147 = Get File Size(file=w462, error in=w465) -> (refnum out=w457:refnum<file>, size (in bytes)=w461:i64, 0:w459:errorcluster)
      n148 = Greater?(x=w461, y=i64 0) -> (0:w466:bool)
      n149 = Set File Position(refnum=w457, from (0:start)=enum16{"start", "end", "current"}."end", error in=w459) -> (refnum out=w456:refnum<file>, error out=w458:errorcluster)  [unwired: 1 out]
      n150 = Select(t=w449, s=w466, f=w451) -> (s? t:f=w463:string)
      n151 = Write to Text File(file (use dialog)=w456, text=w463, error in=w458) -> (error out=w441:errorcluster)  [unwired: 3 out]
    }
    frame #12 {
      n152 = Index Array(array=w473, index (row)=12) -> (element=w472:string[])  [unwired: 1 in]
      n153 = Build Array (concatenate)(w481, w480, w479, w478, w475, w472, w471) -> (w482:string[])
      n154 = Array To Spreadsheet String(delimiter (Tab)=",", array=w483, 3:"" ("format string")) -> (spreadsheet string=w487:string)
      n155 = Array To Spreadsheet String(delimiter (Tab)=",", array=w482, 3:"" ("format string")) -> (spreadsheet string=w484:string)
      n156 = Build Path(base path=w485, name or relative path=w470) -> (appended path=w499:path)
      n157 = Open/Create/Replace File(file path (use dialog)=w499, error in=w477, operation (0:open)=T3."open or create") -> (refnum out=w497:refnum<file>, error out=w500:errorcluster)  [unwired: 4 out]
      n158 = Concatenate Strings(w487, w484) -> (w486:string)
      n159 = Get File Size(file=w497, error in=w500) -> (refnum out=w492:refnum<file>, size (in bytes)=w496:i64, 0:w494:errorcluster)
      n160 = Greater?(x=w496, y=i64 0) -> (0:w501:bool)
      n161 = Set File Position(refnum=w492, from (0:start)=enum16{"start", "end", "current"}."end", error in=w494) -> (refnum out=w491:refnum<file>, error out=w493:errorcluster)  [unwired: 1 out]
      n162 = Select(t=w484, s=w501, f=w486) -> (s? t:f=w498:string)
      n163 = Write to Text File(file (use dialog)=w491, text=w498, error in=w493) -> (error out=w476:errorcluster)  [unwired: 3 out]
    }
    frame #13 {
      n164 = Index Array(array=w507, index (row)=13) -> (element=w508:string[])  [unwired: 1 in]
      n165 = Build Array (concatenate)(w516, w515, w514, w513, w510, w508, w506) -> (w517:string[])
      n166 = Array To Spreadsheet String(delimiter (Tab)=",", array=w518, 3:"" ("format string")) -> (spreadsheet string=w522:string)
      n167 = Array To Spreadsheet String(delimiter (Tab)=",", array=w517, 3:"" ("format string")) -> (spreadsheet string=w519:string)
      n168 = Build Path(base path=w520, name or relative path=w505) -> (appended path=w534:path)
      n169 = Open/Create/Replace File(file path (use dialog)=w534, error in=w512, operation (0:open)=T3."open or create") -> (refnum out=w532:refnum<file>, error out=w535:errorcluster)  [unwired: 4 out]
      n170 = Concatenate Strings(w522, w519) -> (w521:string)
      n171 = Get File Size(file=w532, error in=w535) -> (refnum out=w527:refnum<file>, size (in bytes)=w531:i64, 0:w529:errorcluster)
      n172 = Greater?(x=w531, y=i64 0) -> (0:w536:bool)
      n173 = Set File Position(refnum=w527, from (0:start)=enum16{"start", "end", "current"}."end", error in=w529) -> (refnum out=w526:refnum<file>, error out=w528:errorcluster)  [unwired: 1 out]
      n174 = Select(t=w519, s=w536, f=w521) -> (s? t:f=w533:string)
      n175 = Write to Text File(file (use dialog)=w526, text=w533, error in=w528) -> (error out=w511:errorcluster)  [unwired: 3 out]
    }
    frame #14 {
      n176 = Index Array(array=w543, index (row)=14) -> (element=w542:string[])  [unwired: 1 in]
      n177 = Build Array (concatenate)(w551, w550, w549, w548, w545, w542, w541) -> (w552:string[])
      n178 = Array To Spreadsheet String(delimiter (Tab)=",", array=w553, 3:"" ("format string")) -> (spreadsheet string=w557:string)
      n179 = Array To Spreadsheet String(delimiter (Tab)=",", array=w552, 3:"" ("format string")) -> (spreadsheet string=w554:string)
      n180 = Build Path(base path=w555, name or relative path=w540) -> (appended path=w569:path)
      n181 = Open/Create/Replace File(file path (use dialog)=w569, error in=w547, operation (0:open)=T3."open or create") -> (refnum out=w567:refnum<file>, error out=w570:errorcluster)  [unwired: 4 out]
      n182 = Concatenate Strings(w557, w554) -> (w556:string)
      n183 = Get File Size(file=w567, error in=w570) -> (refnum out=w562:refnum<file>, size (in bytes)=w566:i64, 0:w564:errorcluster)
      n184 = Greater?(x=w566, y=i64 0) -> (0:w571:bool)
      n185 = Set File Position(refnum=w562, from (0:start)=enum16{"start", "end", "current"}."end", error in=w564) -> (refnum out=w561:refnum<file>, error out=w563:errorcluster)  [unwired: 1 out]
      n186 = Select(t=w554, s=w571, f=w556) -> (s? t:f=w568:string)
      n187 = Write to Text File(file (use dialog)=w561, text=w568, error in=w563) -> (error out=w546:errorcluster)  [unwired: 3 out]
    }
    frame #15 {
      n188 = Index Array(array=w578, index (row)=15) -> (element=w577:string[])  [unwired: 1 in]
      n189 = Build Array (concatenate)(w586, w585, w584, w583, w580, w577, w576) -> (w587:string[])
      n190 = Array To Spreadsheet String(delimiter (Tab)=",", array=w588, 3:"" ("format string")) -> (spreadsheet string=w592:string)
      n191 = Array To Spreadsheet String(delimiter (Tab)=",", array=w587, 3:"" ("format string")) -> (spreadsheet string=w589:string)
      n192 = Build Path(base path=w590, name or relative path=w575) -> (appended path=w604:path)
      n193 = Open/Create/Replace File(file path (use dialog)=w604, error in=w582, operation (0:open)=T3."open or create") -> (refnum out=w602:refnum<file>, error out=w605:errorcluster)  [unwired: 4 out]
      n194 = Concatenate Strings(w592, w589) -> (w591:string)
      n195 = Get File Size(file=w602, error in=w605) -> (refnum out=w597:refnum<file>, size (in bytes)=w601:i64, 0:w599:errorcluster)
      n196 = Greater?(x=w601, y=i64 0) -> (0:w606:bool)
      n197 = Set File Position(refnum=w597, from (0:start)=enum16{"start", "end", "current"}."end", error in=w599) -> (refnum out=w596:refnum<file>, error out=w598:errorcluster)  [unwired: 1 out]
      n198 = Select(t=w589, s=w606, f=w591) -> (s? t:f=w603:string)
      n199 = Write to Text File(file (use dialog)=w596, text=w603, error in=w598) -> (error out=w581:errorcluster)  [unwired: 3 out]
    }
  }
  "error out" <- w48
